vi "count rate.vi"() -> ()   [LabVIEW 2014]
uses:
  <vilib>/Platform/TimedLoop/XDataNode/timing_clust.ctl
  <vilib>/Platform/TimedLoop/XDataNode/nitl_modes.ctl
  <vilib>/Platform/TimedLoop/XDataNode/wakeup.ctl
  <vilib>/platform/TimedLoop/XDataNode/XDataNode.xnode
  <vilib>/Platform/TimedLoop/XDataNode/XDNodeRunTimeDep.lvlib
panel:
  out "XY Graph":cluster{i64[], i32[]}(graph)={[0, 1, 2, 3, 4, 5, 6, 7, 8, 9, 10, 11, 12, 13, 14, 15, 16, 17, 18, 19, 20, 21, 22, 23, 24, 25, 26, 27, 28, 29, 30, 31, 32, 33, 34, 35, 36, 37, 38, 39, 40, 41, 42, 43, 44, 45, 46, 47, 48, 49, 50, 51, 52, 53, 54, 55, 56, 57, 58, 59, 60, 61, 62, 63, 64, 65, 66, 67, 68, 69, 70, 71, 72, 73, 74, 75, 76, 77, 78, 79, 80, 81, 82, 83, 84, 85, 86, 87, 88, 89, 90, 91, 92, 93, 94, 95, 96, 97, 98, 99, 100, 101, 102, 103, 104, 105, 106, 107, 108, 109, 110, 111, 112, 113, 114, 115, 116, 117, 118, 119, 120, 121, 122, 123, 124, 125, 126, 127, 128, 129, 130, 131, 132, 133, 134, 135, 136, 137, 138, 139, 140, 141, 142, 143, 144, 145, 146, 147, 148, 149, 150, 151, 152, 153, 154, 155, 156, 157, 158, 159, 160, 161, 162, 163, 164, 165, 166, 167, 168, 169, 170, 171, 172, 173, 174, 175, 176, 177, 178, 179, 180, 181, 182, 183, 184, 185, 186, 187, 188, 189, 190, 191, 192, 193, 194, 195, 196, 197, 198, 199, 200, 201, 202, 203, 204, 205, 206, 207, 208, 209, 210, 211, 212, 213, 214, 215, 216, 217, 218, 219, 220, 221, 222, 223, 224, 225, 226, 227, 228, 229, 230, 231, 232, 233, 234, 235, 236, 237, 238, 239, 240, 241, 242, 243, 244, 245, 246, 247, 248, 249, 250, 251, 252, 253, 254, 255, 256, 257, 258, 259, 260, 261, 262, 263, 264, 265, 266, 267, 268, 269, 270, 271, 272, 273, 274, 275, 276, 277, 278, 279, 280, 281, 282, 283, 284, 285, 286, 287, 288, 289, 290, 291, 292, 293, 294, 295, 296, 297, 298, 299, 300], [0, 75, 86, 72, 76, 79, 69, 66, 83, 71, 77, 89, 72, 85, 73, 68, 70, 68, 83, 74, 76, 59, 63, 80, 69, 62, 71, 69, 59, 65, 72, 59, 65, 61, 71, 68, 52, 67, 49, 60, 73, 48, 54, 58, 70, 69, 68, 56, 51, 69, 66, 50, 50, 58, 44, 58, 59, 44, 44, 48, 59, 61, 56, 52, 60, 55, 49, 43, 51, 47, 53, 62, 41, 40, 44, 41, 46, 48, 51, 48, 42, 49, 43, 45, 46, 48, 49, 64, 39, 52, 40, 42, 32, 26, 42, 45, 38, 46, 35, 33, 27, 29, 44, 40, 38, 32, 37, 46, 41, 31, 38, 30, 24, 33, 33, 23, 30, 36, 31, 42, 34, 32, 36, 39, 26, 32, 34, 28, 22, 31, 41, 24, 22, 28, 20, 35, 30, 24, 34, 27, 30, 33, 26, 20, 28, 30, 31, 31, 19, 24, 23, 24, 21, 23, 22, 27, 19, 29, 17, 30, 30, 31, 28, 24, 24, 21, 25, 21, 22, 18, 19, 26, 21, 19, 24, 20, 17, 19, 19, 14, 23, 19, 20, 20, 16, 15, 13, 15, 17, 14, 15, 23, 14, 20, 22, 23, 14, 14, 19, 13, 14, 17, 9, 16, 13, 17, 16, 15, 17, 17, 14, 15, 12, 9, 12, 14, 21, 24, 16, 14, 13, 18, 23, 13, 7, 14, 10, 14, 13, 19, 8, 14, 15, 8, 15, 12, 10, 12, 11, 9, 17, 10, 8, 15, 14, 11, 10, 16, 12, 18, 12, 12, 19, 11, 8, 20, 16, 15, 9, 12, 7, 9, 9, 9, 8, 16, 8, 12, 12, 16, 7, 14, 10, 12, 13, 11, 4, 10, 13, 10, 8, 11, 19, 13, 11, 12, 10, 6, 6, 7, 8, 7, 8, 13, 10, 8, 18, 5, 10, 12, 13]}
  in  "file path (use dialog)":path=path "C:/Users/eclifton/Documents/GitHub/week8/count_data2.txt"
  in  "Total Time":dbl=300.0
  in  "Time Inc.":i64=1
  out "counts per second":dbl(knob)=13.0 scale=0.0..100.0
  in  "stop":bool
  # "Demo count rate VI for Physics 434"
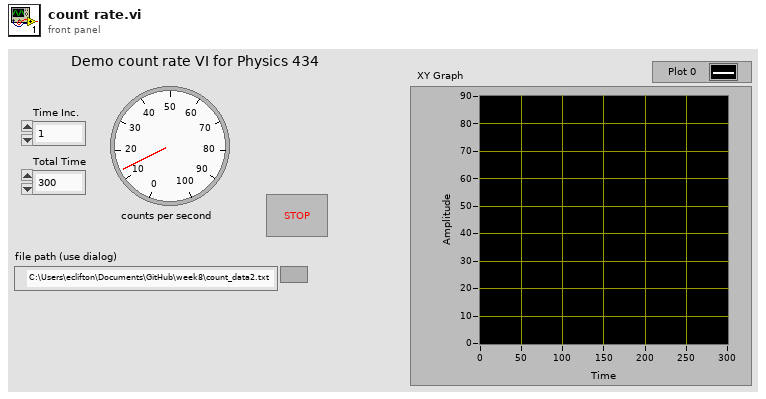
[diagram p1: front panel]
types:
  T1 = typedef "XDNodeRunTimeDep.lvlib/timing_clust.ctl" = cluster{"Expected End [f-1]":u64, "Actual End [f-1]":u64, "Finished Late? [f-1]":bool, "Expected End [i-1]":u64, "Actual End [i-1]":u64, "Finished Late? [i-1]":bool, "Expected Start [i]":u64, "Actual Start [i]":u64, "Expected Start [f]":u64, "Actual Start [f]":u64, "Source Name":string, "Structure Name":string, "Period":i64, "Deadline":i64, "Offset":i64, "Start":i64, "Priority":i32, "Timeout":i32, "Mode":T2, "Wakeup Reason":T3, "Error":errorcluster, "Source Type":string, "Secondary Source Type":string, "Global End Time":u64, "Global Start Time":u64, "Frame Duration":u64, "Iteration Duration":u64, "Assigned CPU":i32, "I/O Scan Engine Mode":u32}
  T2 = typedef "XDNodeRunTimeDep.lvlib/nitl_modes.ctl" = enum32{"No Change", "Process missed periods, maintain original phase", "Discard missed periods, maintain original phase", "Process missed periods, ignore original phase", "Discard missed periods, ignore original phase"}
  T3 = typedef "XDNodeRunTimeDep.lvlib/wakeup.ctl" = enum32{"Normal", "Aborted", "Asynchronous wakeup", "Timing source error", "Timed loop error", "Timeout"}
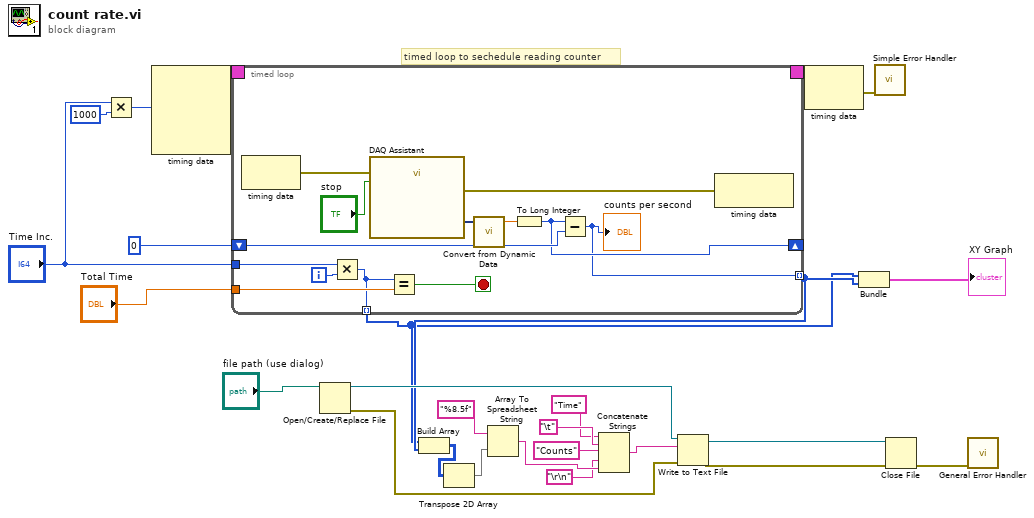
[diagram p0: block diagram]
diagram:
  # "timed loop to sechedule reading counter"
  n1 = Multiply(x="Time Inc.", y=i64 1000) -> (x*y=w20:i64)
  n2 = node-c288(w20) -> (w26:T1)  [unwired: 3 in]
  n3 = timed-loop {
    timing: w26 -> [_]
    timing-out: [_] -> w25
    shift-right: [w29] -> _
    shift-left: 0 -> [w38]
    tunnel: "Total Time" -> [w33]
    tunnel: "Time Inc." -> [w31]
    tunnel: [w27] -> w3 mode=indexing
    tunnel: [w28] -> w2 mode=indexing
    i -> [w32]
    stop <- w30 stop-if-true
    n4 = node-c288() -> (w34:errorcluster)  [unwired: 1 in]
    n5 = Multiply(x=w31, y=w32) -> (x*y=w28:i64)
    n6 = call "DAQ Assistant"("error in"=w34, "stop (F)"="stop") -> ("data"=w39:dynamicdata, "error out"=w35:errorcluster)  [unwired: 14 in, 2 out]
    n7 = Equal?(x=w28, y=w33) -> (x = y?=w30:bool)
    n8 = call "Convert from Dynamic Data"("Dynamic Data Type"=w39) -> ("Scalar"=w36:dbl)  [unwired: 3 in]
    n9 = To Long Integer(number=w36) -> (32bit integer=w29:i32)
    n10 = Subtract(x=w29, y=w38) -> (x-y=w27:i32)
    "counts per second" <- w27
    n11 = node-c288(w35) -> ()  [unwired: 1 out]
  }
  n12 = Open/Create/Replace File(file path (use dialog)="file path (use dialog)") -> (refnum out=w6:refnum<file>, error out=w7:errorcluster)  [unwired: 5 in, 1 out]
  n13 = Build Array(w2, w3) -> (w5:i64[][])
  n14 = Transpose 2D Array(2D array=w5) -> (transposed array=w4:i64[][])
  n15 = Array To Spreadsheet String(array=w4, 3:"%8.5f" ("format string")) -> (spreadsheet string=w16:string)  [unwired: 1 in]
  n16 = Concatenate Strings("Time" ("string"), "\t", "Counts" ("string"), "\r\n", w16) -> (w11:string)
  n17 = Write to Text File(file (use dialog)=w6, text=w11, error in=w7) -> (refnum out=w10:refnum<file>, error out=w9:errorcluster)  [unwired: 1 in, 1 out]
  n18 = node-c288(w25) -> (w23:errorcluster)
  n19 = Bundle(w2, w3) -> (→"XY Graph":cluster{i64[], i32[]})  [unwired: 1 in]
  n20 = call <vilib>:"Simple Error Handler.vi"("error in (no error)"=w23) -> ()  [unwired: 4 in, 5 out]
  n21 = Close File(refnum=w10, error in=w9) -> (error out=w18:errorcluster)  [unwired: 1 out]
  n22 = call <vilib>:"General Error Handler.vi"("error in (no error)"=w18) -> ()  [unwired: 10 in, 5 out]
